vi "Init Bfr Rx - UDP Connection.vi"(8 "error in (no error)":errorcluster, 11 "Rx Loop Data in":T1 {"Data Buffer" format="%016x"}) -> (0 "error out":errorcluster, 3 "Rx Loop Data out":T1 {"Data Buffer" format="%016x"})   [LabVIEW 2016, in "UDP-Custom-Device Engine.lvlib"]
uses:
  UDP-Custom-Device Engine.lvlib
  Types/Engine - Buffered Rx Loop Data.ctl
  Shared/Types/Shared - New Data Options.ctl
  Shared/Types/Shared - Buffer Options.ctl
  Shared/Types/Shared - Header Details.ctl
  Shared/Types/Shared - Buffered.PacketInfo.ctl
  Shared/Types/Shared - Pointer Encoding.ctl
  <vilib>/NI/NIVS Inline Async API/_Data Access Engine/Data Access Engine/Types/Read.DVR.ctl
  <vilib>/NI/NIVS Inline Async API/_Data Access Engine/Access Type Classes/Read/Read.lvclass
  <vilib>/NI/NIVS Inline Async API/_Data Access Engine/Data Access Engine/Types/Write.DVR.ctl
  <vilib>/NI/NIVS Inline Async API/_Data Access Engine/Access Type Classes/Write/Write.lvclass
  Shared/Types/Shared - Duplex Settings.ctl
  <vilib>/Utility/tcp.llb/UDP Multicast Read-Only Open.vi
  Shared/UDP-Custom-Device Shared.lvlib
  <vilib>/NI/NIVS Inline Async API/_Data Access Engine/Data Access Engine/Data Access Engine.lvclass
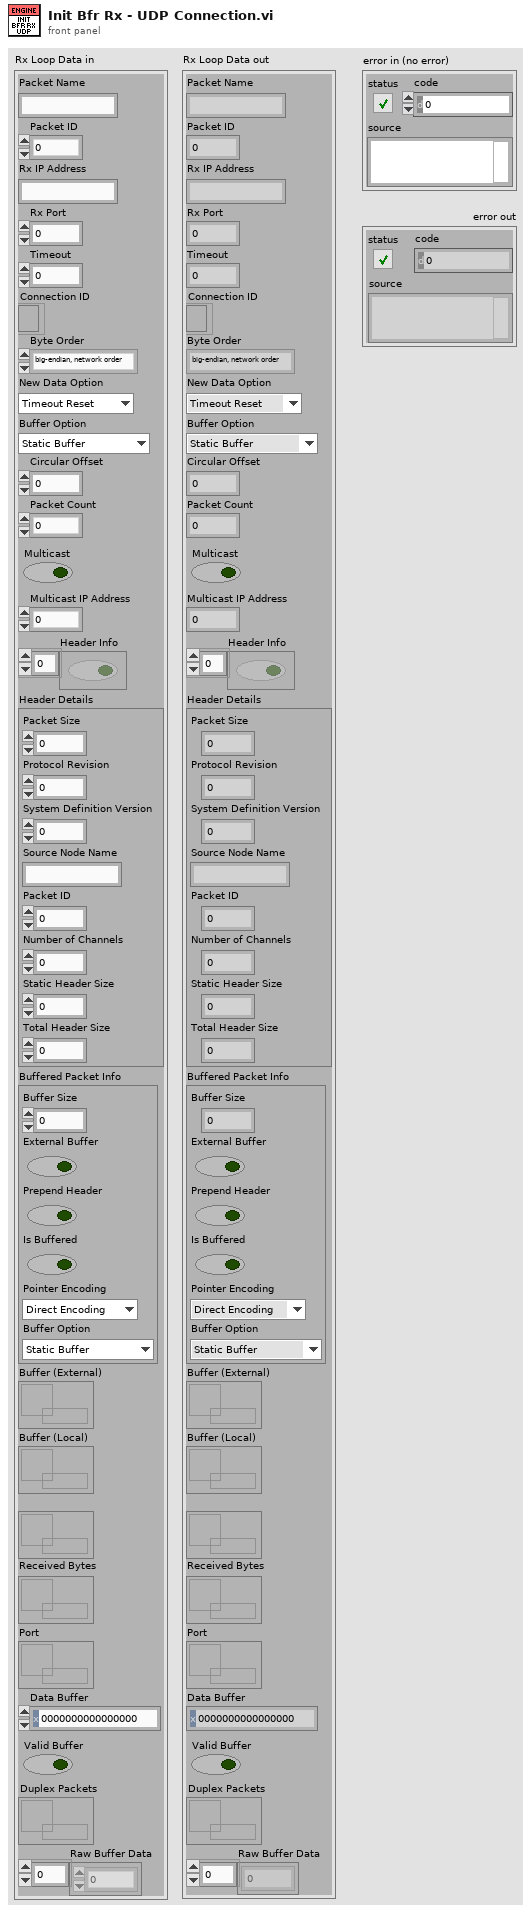
[diagram p1: front panel]
types:
  T1 = typedef "UDP-Custom-Device Engine.lvlib/Engine - Buffered Rx Loop Data.ctl" = cluster{"Packet Name":string, "Packet ID":i32, "Rx IP Address":string, "Rx Port":i32, "Timeout":i32, "Connection ID":refnum<k16>, "Byte Order":enum16{"big-endian, network order", "native, host order", "little-endian"}, "New Data Options":T2, "Buffer Option":T3, "Circular Offset":u64, "Packet Count":dbl, "Multicast":bool, "Multicast IP Address":u32, "Header Info":bool[], "Header Details":T4, "Buffered Packet Info":T5, "Buffer (External)":T7, "Buffer (Local)":T8, "New Data":T8, "Received Bytes":T8, "Port":T8, "Data Buffer":u64, "Valid Buffer":bool, "Duplex Packets":refnum<data-value>, "Raw Buffer Data":u8[]}
  T2 = typedef "UDP-Custom-Device Shared.lvlib/Shared - New Data Options.ctl" = enum16{"Timeout Reset", "Counter"}
  T3 = typedef "UDP-Custom-Device Shared.lvlib/Shared - Buffer Options.ctl" = enum16{"Static Buffer", "Circular Buffer"}
  T4 = typedef "UDP-Custom-Device Shared.lvlib/Shared - Header Details.ctl" = cluster{"Packet Size":u16, "Protocol Revision":u8, "System Definition Version":u64, "Source Node Name":string, "Packet ID":u32, "Number of Channels":u32, "Static Header Size":u16, "Total Header Size":u16}
  T5 = typedef "UDP-Custom-Device Shared.lvlib/Shared - Buffered.PacketInfo.ctl" = cluster{"Buffer Size":i32, "External Buffer":bool, "Prepend Header":bool, "Is Buffered":bool, "Pointer Encoding":T6, "Buffer Option":T3}
  T6 = typedef "UDP-Custom-Device Shared.lvlib/Shared - Pointer Encoding.ctl" = enum16{"Direct Encoding", "Conversion Encoding"}
  T7 = typedef "Data Access Engine.lvlib/Data Access Engine.lvclass/Read.DVR.ctl" = refnum<data-value>
  T8 = typedef "Data Access Engine.lvlib/Data Access Engine.lvclass/Write.DVR.ctl" = refnum<data-value>
  T9 = typedef "UDP-Custom-Device Shared.lvlib/Shared - Duplex Settings.ctl" = cluster{"Transmit Packet ID":i32, "Receive Packet ID":i32, "Multicast":bool, "Multicast Address":string, "IP Address":string, "Port":u16, "TTL":u16, "Duplex Connection":refnum<k16>}
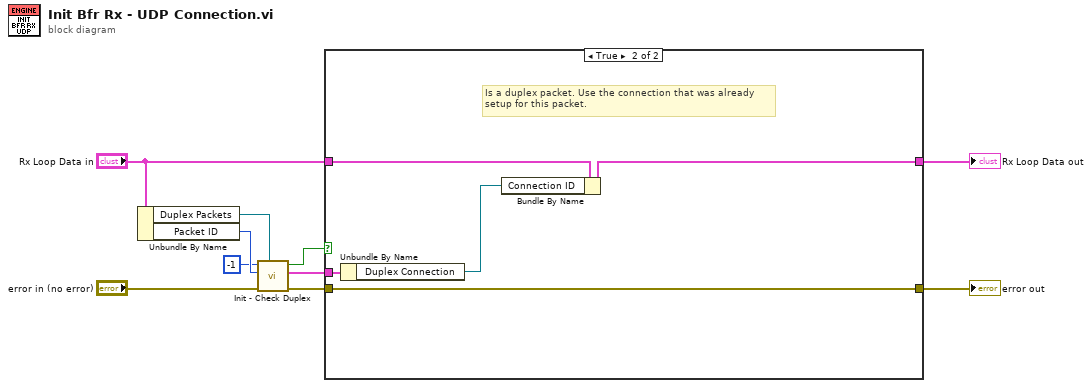
[diagram p0: block diagram]
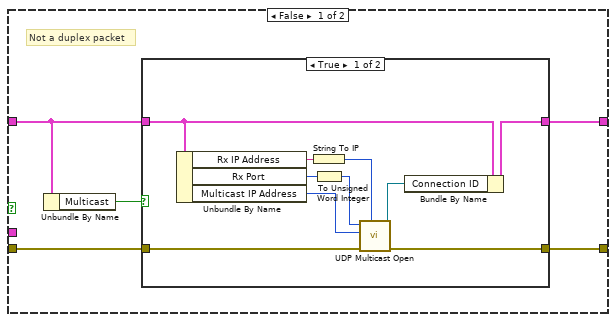
[diagram p2: hidden frame]
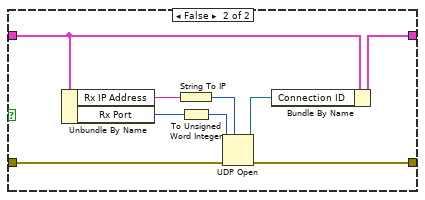
[diagram p3: hidden frame]
diagram:
  n1 = Unbundle By Name("Rx Loop Data in") -> ("Duplex Packets"=w1:refnum<data-value>, "Packet ID"=w8:i32)
  n2 = call "Init - Check Duplex.vi"("Duplex Packets"=w1, "error in (no error)"="error in (no error)", "Receive Packet ID"=w8, "Transmit Packet ID"=-1) -> ("error out"=w5:errorcluster, "Duplex Settings"=w3:T9, "Is Duplex?"=w4:bool)  [unwired: 5 in]
  n3 = case shown="True" w4 {
    tunnel: [w15 w36] -> w10
    tunnel: w5 -> [w14 w35]
    tunnel: [w13 w35] -> w9
    tunnel: "Rx Loop Data in" -> [w12 w37]
    tunnel: w3 -> [_ w38]
    frame False {
      # "Not a duplex packet"
      n4 = Unbundle By Name(w12) -> ("Multicast"=w11:bool)
      n5 = case shown="True" w11 {
        tunnel: w12 -> [w23 w29]
        tunnel: [w22 w28] -> w15
        tunnel: w14 -> [w17 w27]
        tunnel: [w16 w26] -> w13
        frame True {
          n6 = Unbundle By Name(w23) -> ("Rx IP Address"=w25:string, "Rx Port"=w24:i32, "Multicast IP Address"=w19:u32)
          n7 = String To IP(1:w25) -> (0:w21:u32)
          n8 = To Unsigned Word Integer(number=w24) -> (unsigned 16bit integer=w20:u16)
          n9 = call-poly <vilib>:"UDP Multicast Open.vi"("net address"=w21, "error in (no error)"=w17, "multicast addr"=w19, "port"=w20) -> ("error out"=w16:errorcluster, "connection ID"=w18:refnum<k16>)  [unwired: 5 in, 1 out]
          n10 = Bundle By Name(cluster=w23, "Connection ID"=w18) -> (w22:T1)
        }
        frame False {
          n11 = Unbundle By Name(w29) -> ("Rx IP Address"=w31:string, "Rx Port"=w30:i32)
          n12 = String To IP(1:w31) -> (0:w32:u32)
          n13 = To Unsigned Word Integer(number=w30) -> (unsigned 16bit integer=w33:u16)
          n14 = UDP Open(7:w32, 8:w27, 11:w33) -> (port=w34:refnum<k16>, 0:w26:errorcluster)  [unwired: 2 in, 1 out]
          n15 = Bundle By Name(cluster=w29, "Connection ID"=w34) -> (w28:T1)
        }
      }
    }
    frame True {
      # "Is a duplex packet. Use the connection that was already\nsetup for this packet."
      n16 = Unbundle By Name(w38) -> ("Duplex Connection"=w39:refnum<k16>)
      n17 = Bundle By Name(cluster=w37, "Connection ID"=w39) -> (w36:T1)
    }
  }
  "Rx Loop Data out" <- w10
  "error out" <- w9
